vi "Get 1D Time Stamp.vi"(5 "format string (%s)":string="%s", 7 "key description":string, 8 "sections":string[](array[string]), 9 "time stamp":timestamp[](array[timestamp]), 11 "info data":string) -> (0 "sections out":string[](array[string]), 1 "found?":bool, 2 "value":timestamp[](array[timestamp]), 3 "info data out":string)   [LabVIEW 2013, in "infolib.lvlib"]
doc: "Reads horizontal or vertical vector of time stamps. If section is entered it searches the key in the section(s)."
uses:
  infolib.lvlib
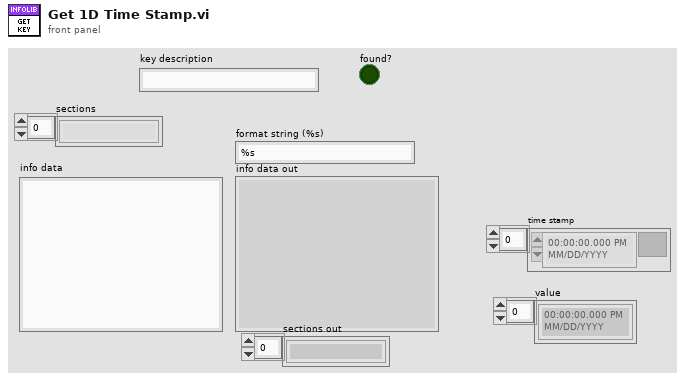
[diagram p1: front panel]
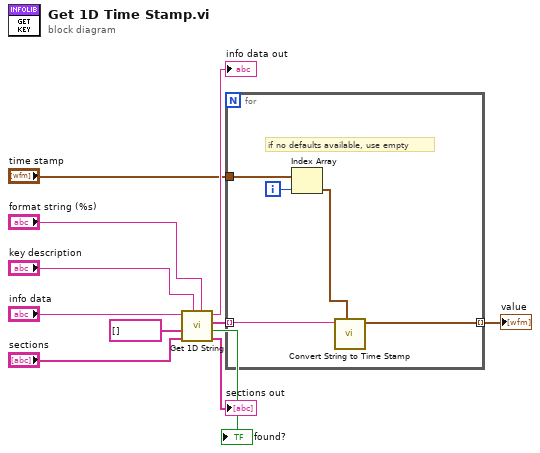
[diagram p0: block diagram]
diagram:
  n1 = call "Get 1D String.vi"("format string (%s)"="format string (%s)", "key description"="key description", "sections"="sections", "string"=string[] [] ("1D string array"), "info data"="info data") -> ("sections out"=→"sections out":string[], "found?"=→"found?":bool, "value"=w5:string[], "info data out"=→"info data out":string)  [unwired: 3 in]
  n2 = for {
    tunnel: w5 -> [w14] mode=indexing
    tunnel: [w12] -> w3 mode=indexing
    tunnel: "time stamp" -> [w16]
    i -> [w15]
    # "if no defaults available, use empty"
    n3 = Index Array(array=w16, index=w15) -> (element=w13:timestamp)
    n4 = call "Convert String to Time Stamp.vi"("default value of time stamp"=w13, "string"=w14) -> ("time stamp out"=w12:timestamp)  [unwired: 9 in]
  }
  "value" <- w3
